vi "Checksum.vi"(4 "String":string, 5 "Check soma?":bool) -> (0 "Checksum?":bool, 1 "Função":u8, 2 "Check":string)   [LabVIEW 2016]
panel:
  out "substring":string
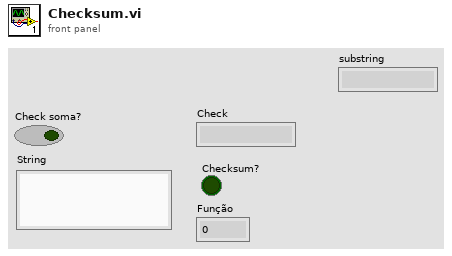
[diagram p1: front panel]
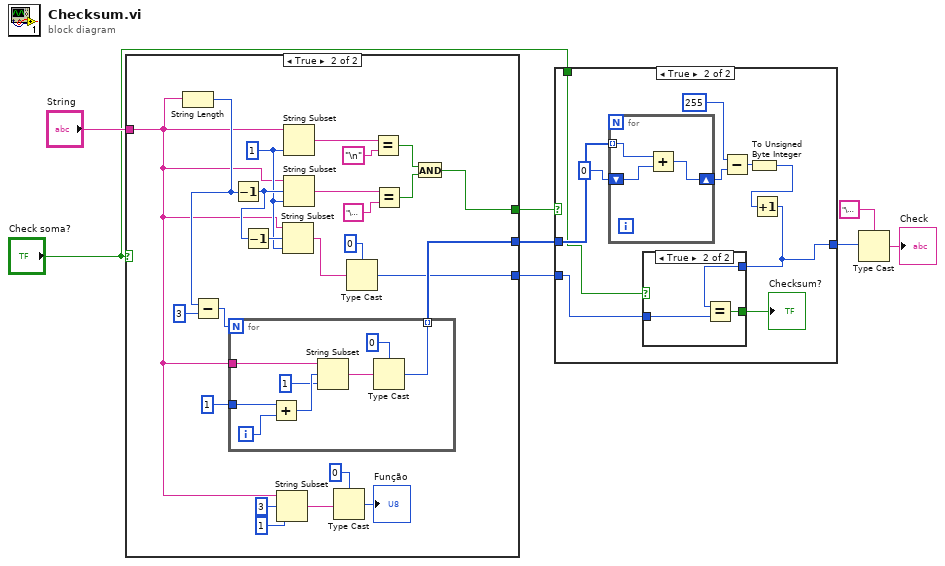
[diagram p0: block diagram]
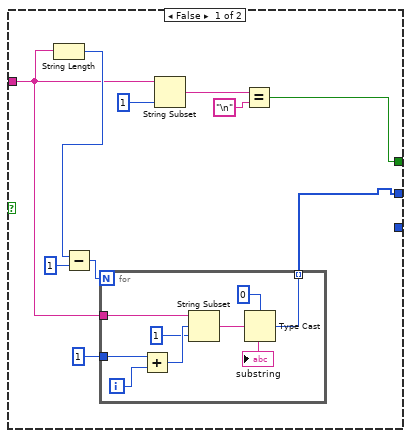
[diagram p2: hidden frame]
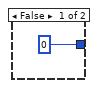
[diagram p3: hidden frame]
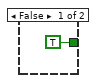
[diagram p4: hidden frame]
diagram:
  n1 = case shown="True" "Check soma?" {
    tunnel: [w9 w44] -> w8
    tunnel: [w11 w39] -> w7
    tunnel: "String" -> [w10 w32]
    tunnel: [_ w33] -> w5
    frame False {
      n2 = String Length(string=w10) -> (length=w15:i32)
      n3 = Subtract(x=w15, y=1 ("length (rest)")) -> (x-y=w13:i32)
      n4 = for {
        N: w13 -> [_]
        tunnel: w10 -> [w26]
        tunnel: 1 ("length (rest)") -> [w25]
        tunnel: [w19] -> w11 mode=indexing
        i -> [w24]
        n5 = Add(x=w25, y=w24) -> (x+y=w23:i32)
        n6 = String Subset(string=w26, offset (0)=w23, length (rest)=1 ("length (rest)")) -> (substring=w21:string)
        "substring" <- w21
        n7 = Type Cast(type=u8 0, x=w21) -> (*(type *) &x=w19:u8)
      }
      n8 = String Subset(string=w10, length (rest)=1 ("length (rest)")) -> (substring=w18:string)  [unwired: 1 in]
      n9 = Equal?(x=w18, y="\n") -> (x = y?=w9:bool)
    }
    frame True {
      w36 = 1 ("length (rest)")
      n10 = String Length(string=w32) -> (length=w42:i32)
      n11 = Subtract(x=w42, y=3 ("length (rest)")) -> (x-y=w40:i32)
      n12 = for {
        N: w40 -> [_]
        tunnel: w32 -> [w58]
        tunnel: 1 ("length (rest)") -> [w57]
        tunnel: [w51] -> w39 mode=indexing
        i -> [w56]
        n13 = Add(x=w57, y=w56) -> (x+y=w55:i32)
        n14 = String Subset(string=w58, offset (0)=w55, length (rest)=1 ("length (rest)")) -> (substring=w53:string)
        n15 = Type Cast(type=u8 0, x=w53) -> (*(type *) &x=w51:u8)
      }
      n16 = Decrement(x=w42) -> (x-1=w38:i32)
      n17 = Decrement(x=w38) -> (x-1=w37:i32)
      n18 = String Subset(string=w32, offset (0)=3, length (rest)=1 ("length (rest)")) -> (substring=w30:string)
      n19 = String Subset(string=w32, offset (0)=w37, length (rest)=w36) -> (substring=w34:string)
      n20 = String Subset(string=w32, length (rest)=w36) -> (substring=w48:string)  [unwired: 1 in]
      n21 = String Subset(string=w32, offset (0)=w38, length (rest)=w36) -> (substring=w49:string)
      n22 = Type Cast(type=u8 0, x=w30) -> (*(type *) &x=→"Função":u8)
      n23 = Type Cast(type=u8 0, x=w34) -> (*(type *) &x=w33:u8)
      n24 = Equal?(x=w48, y="\n") -> (x = y?=w45:bool)
      n25 = Equal?(x=w49, y="\u000f") -> (x = y?=w46:bool)
      n26 = And(x=w45, y=w46) -> (x .and. y?=w44:bool)
    }
  }
  n27 = case shown="True" w8 {
    tunnel: w7 -> [_ w69]
    tunnel: w5 -> [_ w67]
    tunnel: [u8 0 w61] -> w3
    tunnel: "Check soma?" -> [_ w60]
    frame False {
    }
    frame True {
      n28 = for {
        tunnel: w69 -> [w76] mode=indexing
        shift-right: [w75] -> w65
        shift-left: u16 0 -> [w74]
        n29 = Add(x=w76, y=w74) -> (x+y=w75:u16)
      }
      n30 = Subtract(x=u8 255, y=w65) -> (x-y=w63:u16)
      n31 = To Unsigned Byte Integer(number=w63) -> (unsigned 8bit integer=w62:u8)
      n32 = Increment(x=w62) -> (x+1=w61:u8)
      n33 = case shown="True" w60 {
        tunnel: w67 -> [_ w73]
        tunnel: [TRUE w72] -> w66
        tunnel: w61 -> [_ w71]
        frame False {
        }
        frame True {
          n34 = Equal?(x=w71, y=w73) -> (x = y?=w72:bool)
        }
      }
      "Checksum?" <- w66
    }
  }
  n35 = Type Cast(type="\u000f", x=w3) -> (*(type *) &x=→"Check":string)
